vi "HW1_Control.vi"(0 "VISA resource name":refnum<visa-resource-name>="COM1", 1 "baud rate":u32=9600, 2 "data bits":u16=8 min=5 max=8 step=1, 3 "parity":u16(ring) items=["None", "Odd", "Even", "Mark", "Space"], 4 "stop bits":u16(ring)=10 items=["1.0"=10, "1.5"=15, "2.0"=20], 6 "read":bool=TRUE, 7 "flow control":u16(ring) items=["None"=0, "XON/XOFF"=1, "RTS/CTS"=2, "DTR/DSR"=4]) -> (9 "read string":string, 10 "bytes read":u32)   [LabVIEW 2010]
doc: "The Basic Serial Read and Write example performs a Serial Port Read, a Serial Port Write, or a combination of these actions. The user selects the actions (read or write) on the front panel. If both are selected, the VI will write the data first, read data, and then close the VISA session that is opened to the port. This VI will wait until the specified number of bytes is received at the port or until a termination character is read.\n\nINSTRUCTIONS:\n1) Select the serial resource and configuration parameters (baud rate, data bits, parity, stop bits, flow control).\n2) Select the operations to be performed. \n3) Connect the serial port to your device. If no device is available, perform a loopback test by doing one of the following. Short pins 2 and 3 on a RS-232 cable or short pin 4 to pin 8 and pin 5 to pin 9 on a RS-485/422 cable. \n4) Run the VI to see the data read. (The \"read string\" will match the \"string to write\" if a loopback test was performed.)\n\nNote: The parameters set for the serial port must match the parameters of the connected instrument or device. In this example, the bytes to read parameter specifies the number of bytes that the serial port reads. If there were more bytes at the port than the number specified in bytes to read, those bytes would not be read. Also, if you specify to read more bytes than the number of bytes actually read, you might receive a timeout error message.\n\nOn the block diagram, the Configure Serial Port VI sets the configuration parameters. The front panel displays the controls used to configure the basic parameters, such as baud rate, data bits, and parity. Constants configure the other parameters the user probably does not need set. After the VISA Configure Serial Port VI opens the VISA session and configures the port, the VI passes the VISA resource name to other VIs that perform operations on that VISA resource. The VISA Write function sends a command to the serial device and the VISA Read function returns data based on the command. The VISA Close function then closes the reference to the serial device. It is important to close the reference; otherwise communication through with that port through protocols other than VISA might not be possible."
uses:
  <vilib>/Instr/_visa.llb/VISA Configure Serial Port (Instr).vi
panel:
  in  "On 8":bool
  in  "Off 8":bool
  in  "On 7":bool
  in  "Off 7":bool
  in  "On 6":bool
  in  "Off 6":bool
  in  "On 5":bool
  in  "Off 5":bool
  in  "On 4":bool
  in  "Off 4":bool
  in  "On 3":bool
  in  "Off 3":bool
  in  "On 2":bool
  in  "Off 2":bool
  in  "stop":bool
  in  "On":bool
  in  "Off":bool
  in  "delay before read (ms)":u32=500
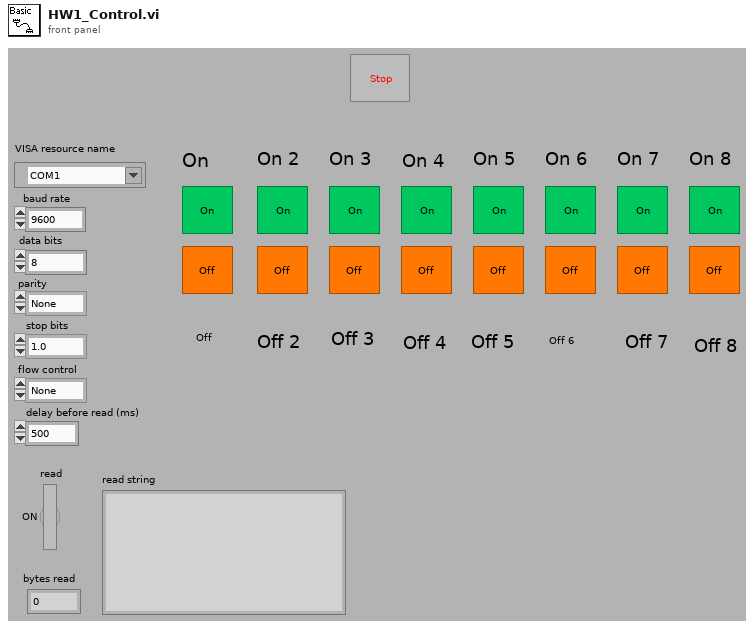
[diagram p1: front panel]
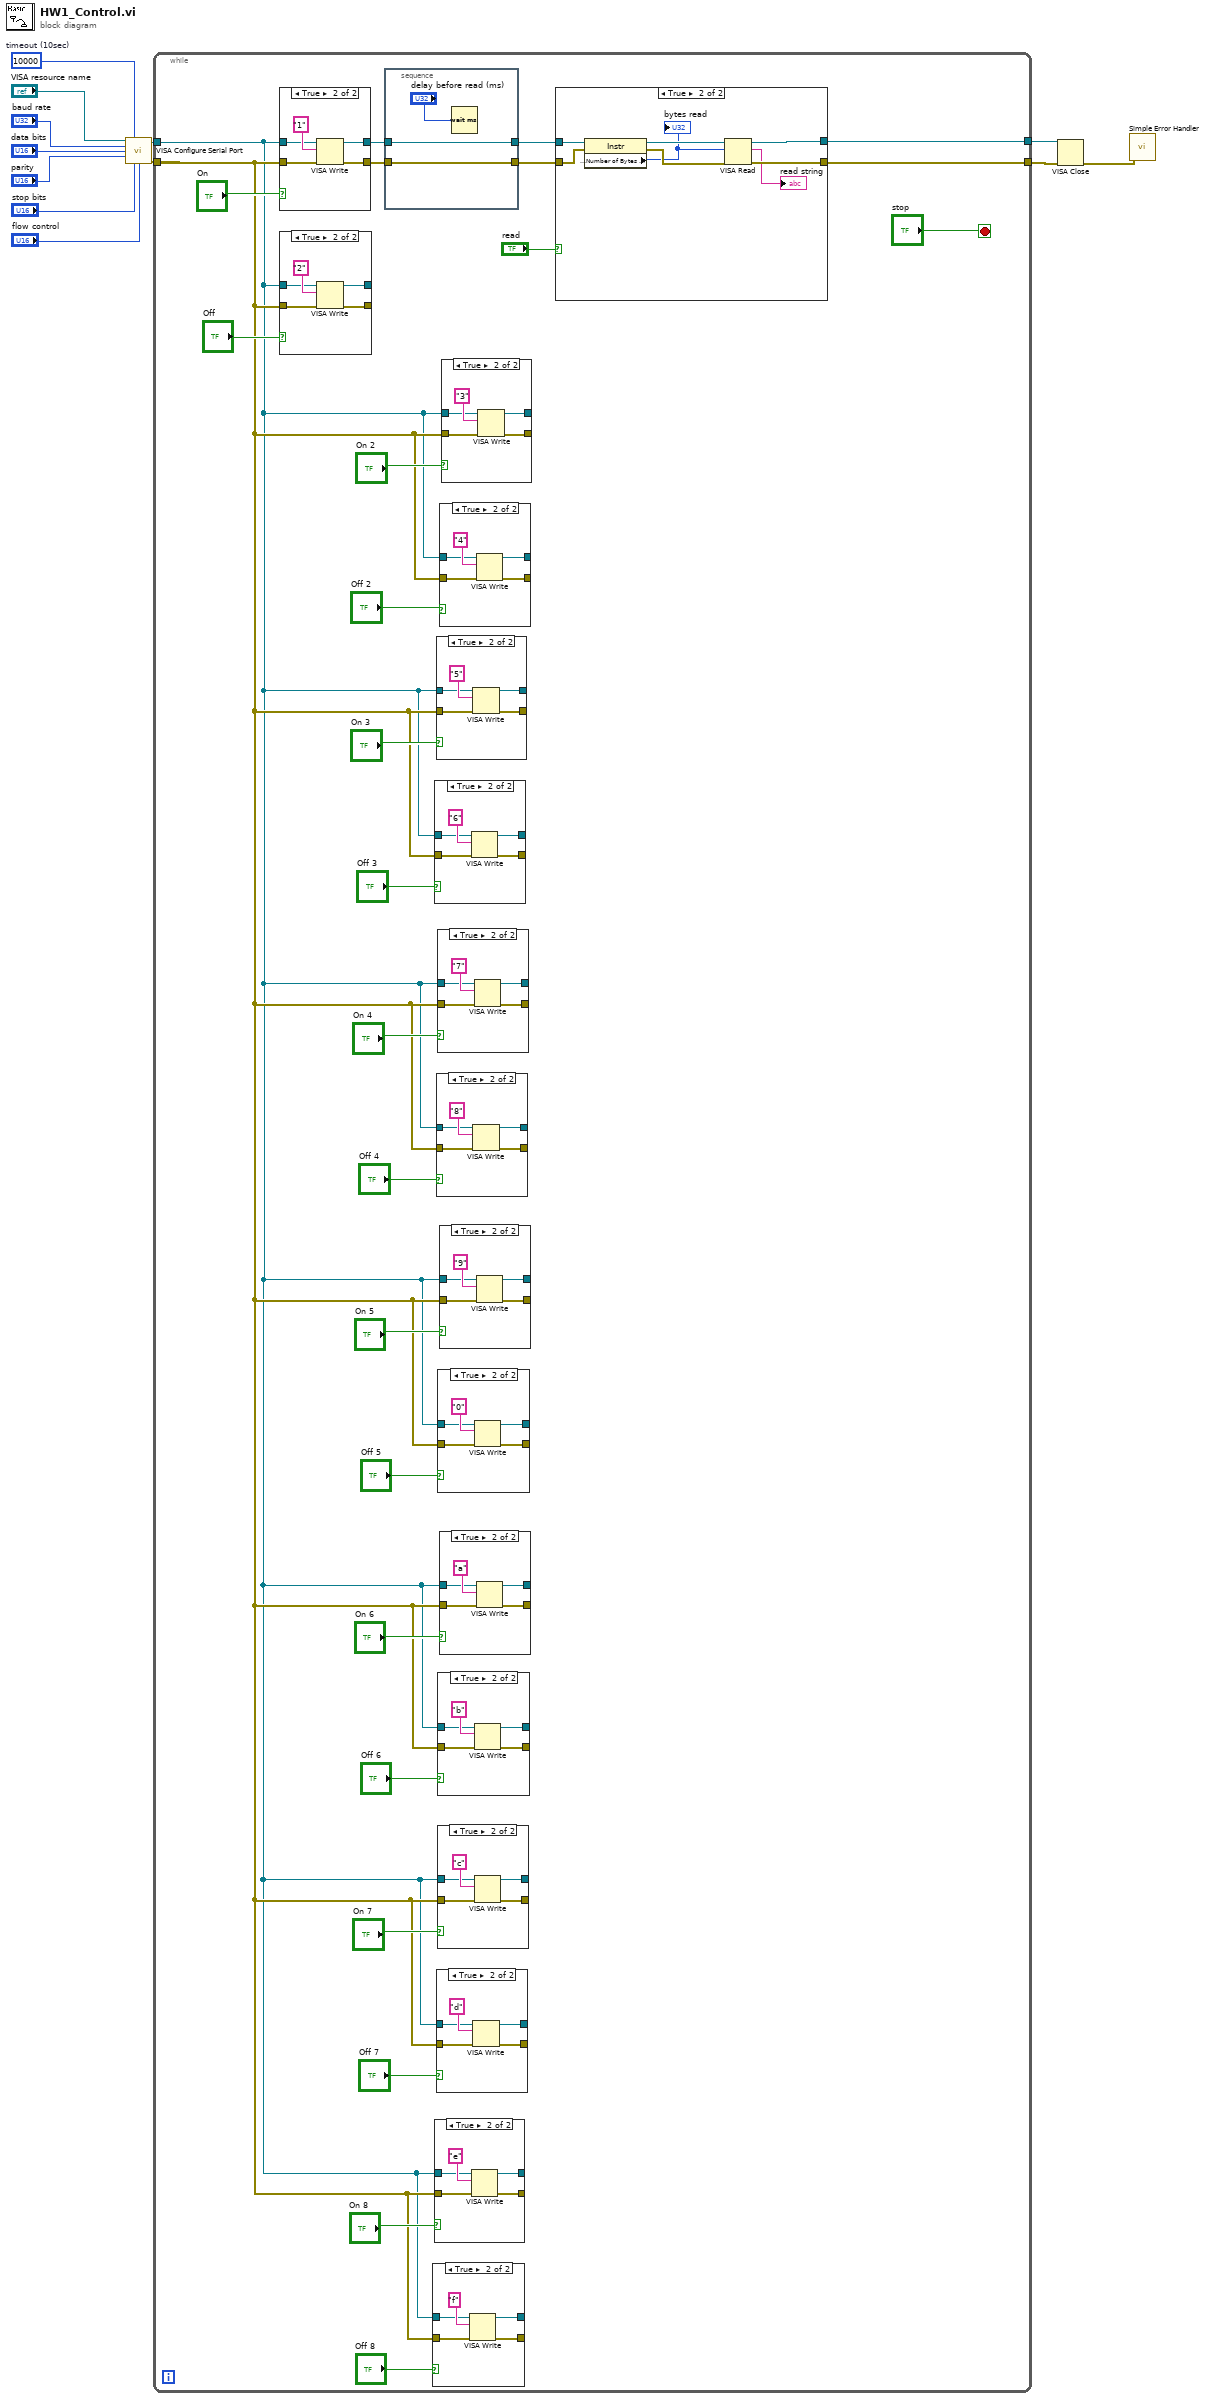
[diagram p0: block diagram]
diagram:
  w8 = u32 10000  # timeout (10sec)
  n1 = call-poly "VISA Configure Serial Port"("VISA resource name"="VISA resource name", "timeout (10sec)"=w8, "baud rate (9600)"="baud rate", "data bits (8)"="data bits", "parity (0:none)"="parity", "stop bits (10: 1 bit)"="stop bits", "flow control (0:none)"="flow control") -> ("VISA resource name out"=w1:refnum<visa-resource-name>, "error out"=w2:errorcluster)  [unwired: 2 in, 5 out]
  n2 = while {
    tunnel: [w30] -> w4
    tunnel: [w29] -> w3
    tunnel: w2 -> [w14]
    tunnel: w1 -> [w13]
    stop <- "stop" stop-if-true
    n3 = case shown="True" "On" {
      tunnel: [w148 w153] -> w32
      tunnel: w13 -> [w147 w151]
      tunnel: w14 -> [w148 w150]
      tunnel: [w147 w149] -> w34
      frame False {
      }
      frame True {
        n4 = VISA Write(VISA resource name=w151, write buffer="1" ("string to write"), error in (no error)=w150) -> (VISA resource name out=w149:refnum<visa-resource-name>, error out=w153:errorcluster)  [unwired: 1 out]
      }
    }
    n5 = case shown="True" "Off" {
      tunnel: [w138 w143] -> _
      tunnel: w13 -> [w137 w141]
      tunnel: w14 -> [w138 w140]
      tunnel: [w137 w139] -> _
      frame False {
      }
      frame True {
        n6 = VISA Write(VISA resource name=w141, write buffer="2" ("string to write"), error in (no error)=w140) -> (VISA resource name out=w139:refnum<visa-resource-name>, error out=w143:errorcluster)  [unwired: 1 out]
      }
    }
    n7 = stacked-sequence {
      tunnel: w32 -> [w146]
      tunnel: [w146] -> w33
      tunnel: w34 -> [w145]
      tunnel: [w145] -> w35
      frame #0 {
        n8 = Wait (ms)(milliseconds to wait="delay before read (ms)") -> ()  [unwired: 1 out]
      }
    }
    n9 = case shown="True" "Off 8" {
      tunnel: [w40 w45] -> _
      tunnel: w13 -> [w39 w43]
      tunnel: w14 -> [w40 w42]
      tunnel: [w39 w41] -> _
      frame False {
      }
      frame True {
        n10 = VISA Write(VISA resource name=w43, write buffer="f" ("string to write"), error in (no error)=w42) -> (VISA resource name out=w41:refnum<visa-resource-name>, error out=w45:errorcluster)  [unwired: 1 out]
      }
    }
    n11 = case shown="True" "Off 3" {
      tunnel: [w110 w115] -> _
      tunnel: w13 -> [w109 w113]
      tunnel: w14 -> [w110 w112]
      tunnel: [w109 w111] -> _
      frame False {
      }
      frame True {
        n12 = VISA Write(VISA resource name=w113, write buffer="6" ("string to write"), error in (no error)=w112) -> (VISA resource name out=w111:refnum<visa-resource-name>, error out=w115:errorcluster)  [unwired: 1 out]
      }
    }
    n13 = case shown="True" "On 8" {
      tunnel: [w47 w52] -> _
      tunnel: w13 -> [w46 w50]
      tunnel: w14 -> [w47 w49]
      tunnel: [w46 w48] -> _
      frame False {
      }
      frame True {
        n14 = VISA Write(VISA resource name=w50, write buffer="e" ("string to write"), error in (no error)=w49) -> (VISA resource name out=w48:refnum<visa-resource-name>, error out=w52:errorcluster)  [unwired: 1 out]
      }
    }
    n15 = case shown="True" "On 3" {
      tunnel: [w117 w122] -> _
      tunnel: w13 -> [w116 w120]
      tunnel: w14 -> [w117 w119]
      tunnel: [w116 w118] -> _
      frame False {
      }
      frame True {
        n16 = VISA Write(VISA resource name=w120, write buffer="5" ("string to write"), error in (no error)=w119) -> (VISA resource name out=w118:refnum<visa-resource-name>, error out=w122:errorcluster)  [unwired: 1 out]
      }
    }
    n17 = case shown="True" "Off 4" {
      tunnel: [w96 w101] -> _
      tunnel: w13 -> [w95 w99]
      tunnel: w14 -> [w96 w98]
      tunnel: [w95 w97] -> _
      frame False {
      }
      frame True {
        n18 = VISA Write(VISA resource name=w99, write buffer="8" ("string to write"), error in (no error)=w98) -> (VISA resource name out=w97:refnum<visa-resource-name>, error out=w101:errorcluster)  [unwired: 1 out]
      }
    }
    n19 = case shown="True" "Off 7" {
      tunnel: [w54 w59] -> _
      tunnel: w13 -> [w53 w57]
      tunnel: w14 -> [w54 w56]
      tunnel: [w53 w55] -> _
      frame False {
      }
      frame True {
        n20 = VISA Write(VISA resource name=w57, write buffer="d" ("string to write"), error in (no error)=w56) -> (VISA resource name out=w55:refnum<visa-resource-name>, error out=w59:errorcluster)  [unwired: 1 out]
      }
    }
    n21 = case shown="True" "On 4" {
      tunnel: [w103 w108] -> _
      tunnel: w13 -> [w102 w106]
      tunnel: w14 -> [w103 w105]
      tunnel: [w102 w104] -> _
      frame False {
      }
      frame True {
        n22 = VISA Write(VISA resource name=w106, write buffer="7" ("string to write"), error in (no error)=w105) -> (VISA resource name out=w104:refnum<visa-resource-name>, error out=w108:errorcluster)  [unwired: 1 out]
      }
    }
    n23 = case shown="True" "Off 5" {
      tunnel: [w82 w87] -> _
      tunnel: w13 -> [w81 w85]
      tunnel: w14 -> [w82 w84]
      tunnel: [w81 w83] -> _
      frame False {
      }
      frame True {
        n24 = VISA Write(VISA resource name=w85, write buffer="0" ("string to write"), error in (no error)=w84) -> (VISA resource name out=w83:refnum<visa-resource-name>, error out=w87:errorcluster)  [unwired: 1 out]
      }
    }
    n25 = case shown="True" "Off 6" {
      tunnel: [w68 w73] -> _
      tunnel: w13 -> [w67 w71]
      tunnel: w14 -> [w68 w70]
      tunnel: [w67 w69] -> _
      frame False {
      }
      frame True {
        n26 = VISA Write(VISA resource name=w71, write buffer="b" ("string to write"), error in (no error)=w70) -> (VISA resource name out=w69:refnum<visa-resource-name>, error out=w73:errorcluster)  [unwired: 1 out]
      }
    }
    n27 = case shown="True" "On 7" {
      tunnel: [w61 w66] -> _
      tunnel: w13 -> [w60 w64]
      tunnel: w14 -> [w61 w63]
      tunnel: [w60 w62] -> _
      frame False {
      }
      frame True {
        n28 = VISA Write(VISA resource name=w64, write buffer="c" ("string to write"), error in (no error)=w63) -> (VISA resource name out=w62:refnum<visa-resource-name>, error out=w66:errorcluster)  [unwired: 1 out]
      }
    }
    n29 = case shown="True" "Off 2" {
      tunnel: [w124 w129] -> _
      tunnel: w13 -> [w123 w127]
      tunnel: w14 -> [w124 w126]
      tunnel: [w123 w125] -> _
      frame False {
      }
      frame True {
        n30 = VISA Write(VISA resource name=w127, write buffer="4" ("string to write"), error in (no error)=w126) -> (VISA resource name out=w125:refnum<visa-resource-name>, error out=w129:errorcluster)  [unwired: 1 out]
      }
    }
    n31 = case shown="True" "On 5" {
      tunnel: [w89 w94] -> _
      tunnel: w13 -> [w88 w92]
      tunnel: w14 -> [w89 w91]
      tunnel: [w88 w90] -> _
      frame False {
      }
      frame True {
        n32 = VISA Write(VISA resource name=w92, write buffer="9" ("string to write"), error in (no error)=w91) -> (VISA resource name out=w90:refnum<visa-resource-name>, error out=w94:errorcluster)  [unwired: 1 out]
      }
    }
    n33 = case shown="True" "On 6" {
      tunnel: [w75 w80] -> _
      tunnel: w13 -> [w74 w78]
      tunnel: w14 -> [w75 w77]
      tunnel: [w74 w76] -> _
      frame False {
      }
      frame True {
        n34 = VISA Write(VISA resource name=w78, write buffer="a" ("string to write"), error in (no error)=w77) -> (VISA resource name out=w76:refnum<visa-resource-name>, error out=w80:errorcluster)  [unwired: 1 out]
      }
    }
    n35 = case shown="True" "On 2" {
      tunnel: [w131 w136] -> _
      tunnel: w13 -> [w130 w134]
      tunnel: w14 -> [w131 w133]
      tunnel: [w130 w132] -> _
      frame False {
      }
      frame True {
        n36 = VISA Write(VISA resource name=w134, write buffer="3" ("string to write"), error in (no error)=w133) -> (VISA resource name out=w132:refnum<visa-resource-name>, error out=w136:errorcluster)  [unwired: 1 out]
      }
    }
    n37 = case shown="True" "read" {
      tunnel: w33 -> [w155 w159]
      tunnel: [w155 w163] -> w29
      tunnel: [w154 w162] -> w30
      tunnel: w35 -> [w154 w161]
      frame False {
        (unwired) 0
      }
      frame True {
        n38 = property class="Instr"(reference=w161, error in=w159) -> (reference out=w160:refnum<visa-resource-name>, error out=w158:errorcluster, "Serial Settings:Number of Bytes at Serial Port"=w157:u32)
        "bytes read" <- w157
        n39 = VISA Read(VISA resource name=w160, byte count=w157, error in (no error)=w158) -> (VISA resource name out=w162:refnum<visa-resource-name>, read buffer=→"read string":string, error out=w163:errorcluster)  [unwired: 1 out]
      }
    }
  }
  n40 = VISA Close(VISA resource name=w4, error in (no error)=w3) -> (error out=w10:errorcluster)
  n41 = call <vilib>:"Simple Error Handler.vi"("error in (no error)"=w10) -> ()  [unwired: 1 in, 8 out]
